vi "FilePathToSaveFGV.vi"(6 "FilePathToSaveAction":T1=enum."Get file path", 8 "ErrorIn":errorcluster, 9 "FilesNames":string="pomiar", 10 "Index":u32, 11 "DirPath":path) -> (0 "ErrorOut":errorcluster, 1 "FileNamesOut":string, 2 "IndexOut":u32, 3 "File path":path)   [LabVIEW 2019]
uses:
  FilePathToSaveAction.ctl
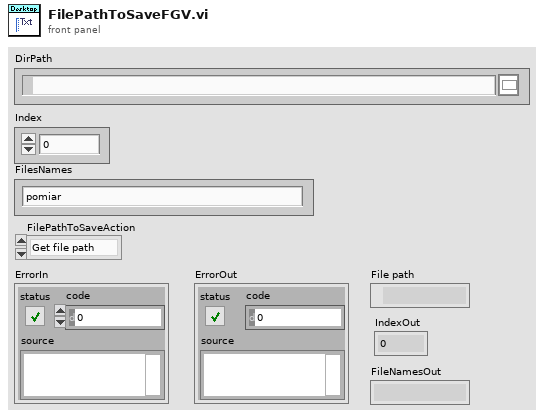
[diagram p1: front panel]
types:
  T1 = typedef "FilePathToSaveAction.ctl" = enum16{"Build new path", "Update index", "Get file path", "Get current settings"}
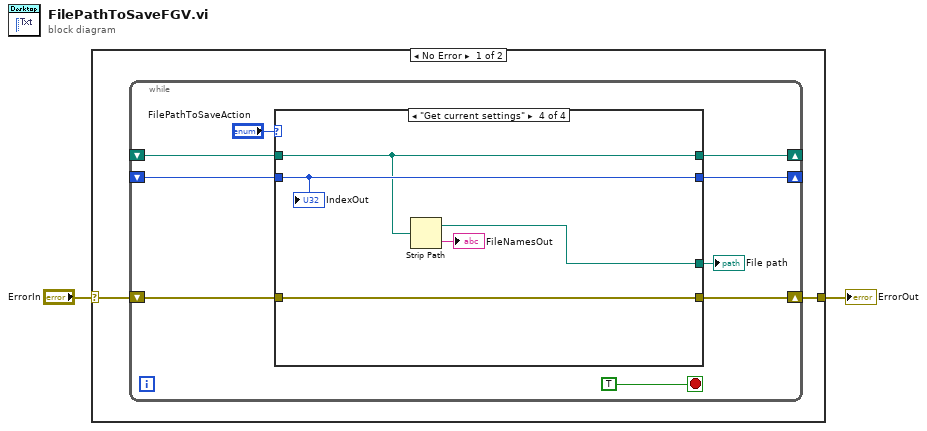
[diagram p0: block diagram]
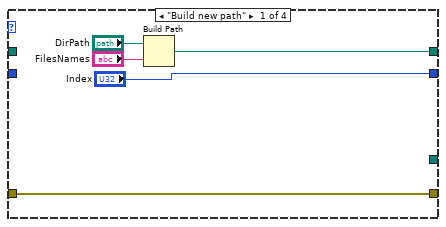
[diagram p2: hidden frame]
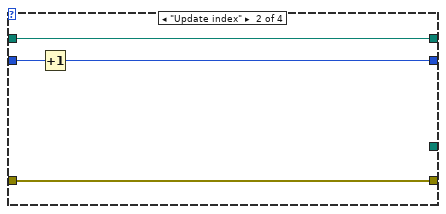
[diagram p3: hidden frame]
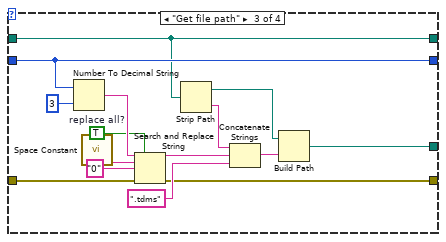
[diagram p4: hidden frame]
diagram:
  n1 = case shown="No Error" "ErrorIn" {
    selector: "ErrorIn" -> [w4 w43]
    tunnel: [w3 w43] -> w1
    frame No Error {
      n2 = while {
        shift-right: [w11] -> w3
        shift-left: w4 -> [w12]
        shift-right: [w8] -> _
        shift-left: _ -> [w9]
        shift-right: [w7] -> _
        shift-left: _ -> [w6]
        stop <- TRUE stop-if-true
        n3 = case shown="\"Get current settings\"" "FilePathToSaveAction" {
          tunnel: w12 -> [w15 w22 w30 w41]
          tunnel: [w15 w22 w28 w41] -> w11
          tunnel: w9 -> [_ w21 w27 w40]
          tunnel: [w17 w21 w27 w40] -> w8
          tunnel: ["Index" w19 w29 w42] -> w7
          tunnel: w6 -> [_ w20 w29 w42]
          tunnel: [_ _ w23 w39] -> w5
          frame "Build new path" {
            n4 = Build Path(base path="DirPath", name or relative path="FilesNames") -> (appended path=w17:path)
          }
          frame "Update index" {
            n5 = Increment(x=w20) -> (x+1=w19:u32)
          }
          frame "Get file path" {
            w33 = TRUE  # replace all?
            n6 = Number To Decimal String(number=w29, width (-)=i16 3) -> (decimal integer string=w35:string)
            n7 = call <vilib>:"Space Constant.vi"() -> ("String"=w36:string)
            n8 = Search and Replace String(replace all?=w33, input string=w35, search string=w36, replace string="0" ("replace string (\"\")"), error in=w30) -> (result string=w37:string, error out=w28:errorcluster)  [unwired: 3 in, 2 out]
            n9 = Strip Path(path=w27) -> (stripped path=w24:path, name=w26:string)
            n10 = Concatenate Strings(w26, w37, ".tdms" ("string")) -> (w25:string)
            n11 = Build Path(base path=w24, name or relative path=w25) -> (appended path=w23:path)
          }
          frame "Get current settings" {
            n12 = Strip Path(path=w40) -> (stripped path=w39:path, name=→"FileNamesOut":string)
            "IndexOut" <- w42
          }
        }
        "File path" <- w5
      }
    }
    frame Error {
    }
  }
  "ErrorOut" <- w1
